vi "ParseInputStream.vi"(10 "EscapePattern":T1, 11 "Data In":u8[](array[numeric])) -> (3 "Array":T2[](array[typedef]))   [LabVIEW 2009]
uses:
  Packet.ctl
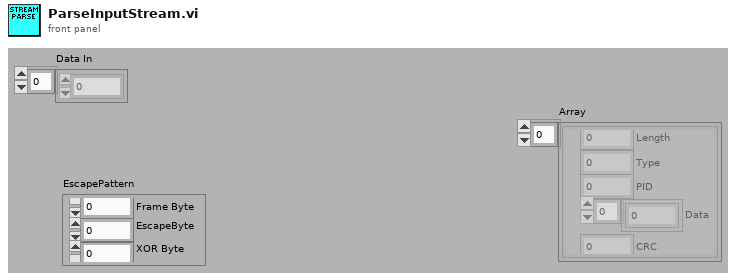
[diagram p1: front panel]
types:
  T1 = cluster{"Frame Byte":u8, "EscapeByte":u8, "XOR Byte":u8}
  T2 = typedef "Packet.ctl" = cluster{"Length":u8, "Type":u8, "PID":u8, "Data":u8[], "CRC":u8}
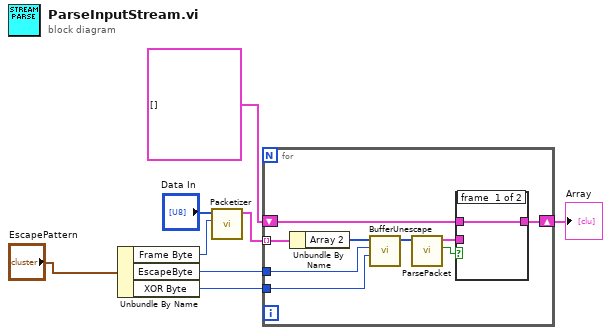
[diagram p0: block diagram]
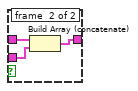
[diagram p2: hidden frame]
diagram:
  n1 = Unbundle By Name("EscapePattern") -> ("Frame Byte"=w4:u8, "EscapeByte"=w3:u8, "XOR Byte"=w2:u8)
  n2 = call "Packetizer.vi"("TokenByte"=w4, "Data In"="Data In") -> ("Tokens"=w8:cluster{"Array 2":u8[]}[])  [unwired: 9 in]
  n3 = for {
    tunnel: w8 -> [w17] mode=indexing
    shift-right: [w11] -> w6
    shift-left: T2[] [] ("Array") -> [w12]
    tunnel: w3 -> [w10]
    tunnel: w2 -> [w9]
    n4 = Unbundle By Name(w17) -> ("Array 2"=w16:u8[])
    n5 = call "BufferUnescape.vi"("XOR Byte"=w9, "EscapeByte"=w10, "Buffer In"=w16) -> ("Buffer Out"=w15:u8[])  [unwired: 8 in]
    n6 = call "ParsePacket.vi"("Buffer"=w15) -> ("Ok?"=w14:bool, "Packet"=w13:T2)  [unwired: 9 in]
    n7 = case shown="False" w14 {
      tunnel: w13 -> [_ w21]
      tunnel: w12 -> [w18 w20]
      tunnel: [w18 w19] -> w11
      frame #0 {
      }
      frame #1 {
        n8 = Build Array (concatenate)(w20, w21) -> (w19:T2[])
      }
    }
  }
  "Array" <- w6
